vi "AE Paper.vi"(0 "error in (no error)":errorcluster, 1 "Message Queue in":T2, 2 "Events":dbl, 3 "Action Events":T1=enum."Init") -> (7 "error out":errorcluster, 9 "Event Increase":dbl)   [LabVIEW 2013, in "main.lvlib"]
uses:
  main.lvlib
  Components/Dependencies.llb/amc_Message Queue.ctl
  Components/Dependencies.llb/amc_Message.ctl
  <vilib>/FTP/util/Keyed Array.ctl
  Controls/Enum Paper Action Events.ctl
  Components/Dependencies.llb/TLB_Dependencies.lvlib
  <vilib>/FTP/NI_FTP.lvlib
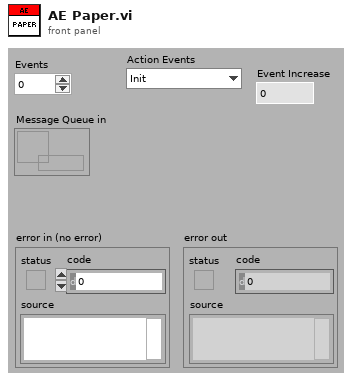
[diagram p1: front panel]
types:
  T1 = typedef "main.lvlib/Enum Paper Action Events.ctl" = enum16{"Paper State", "Init"}
  T2 = typedef "main.lvlib/TLB_Dependencies.lvlib/amc_Message Queue.ctl" = refnum<queue>
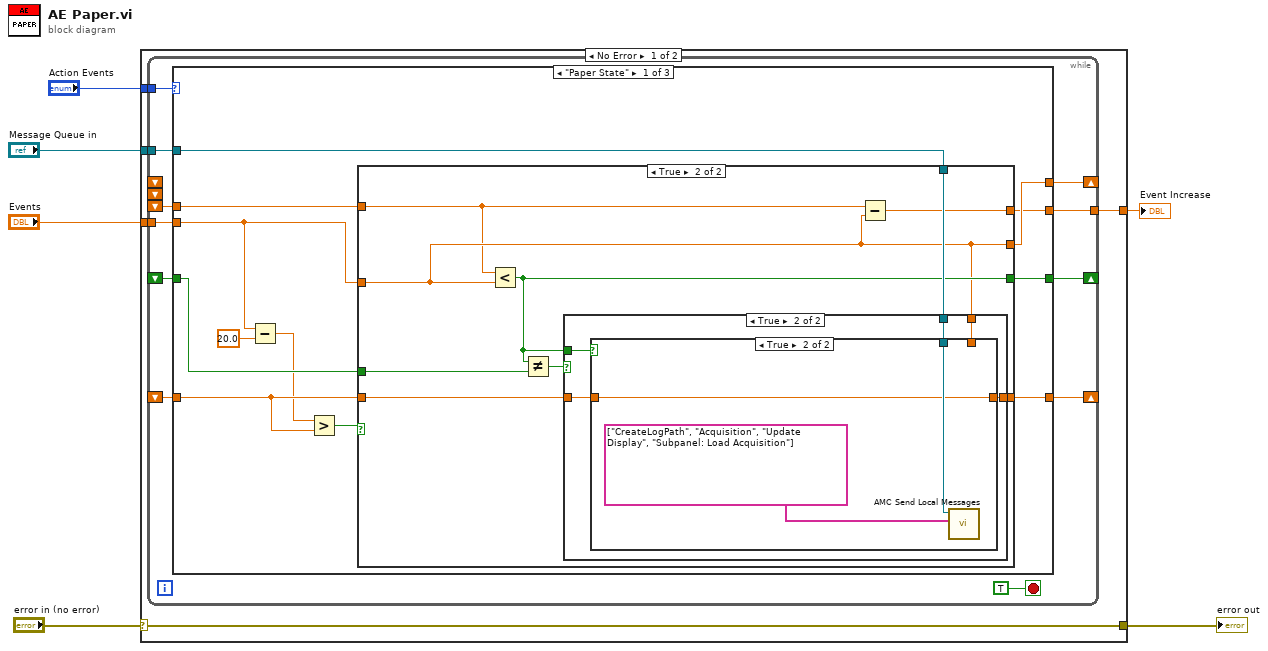
[diagram p0: block diagram]
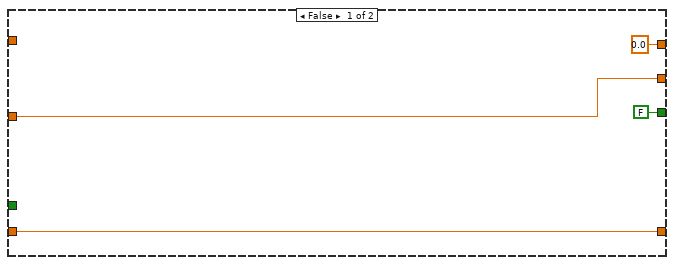
[diagram p2: hidden frame]
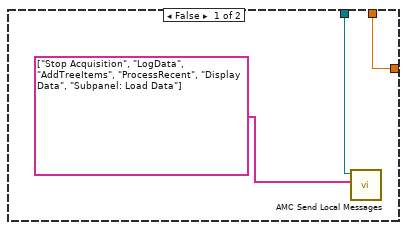
[diagram p4: hidden frame]
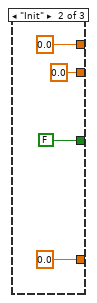
[diagram p5: hidden frame]
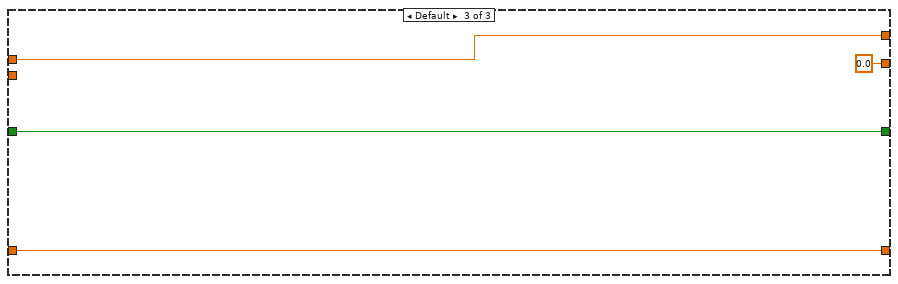
[diagram p6: hidden frame]
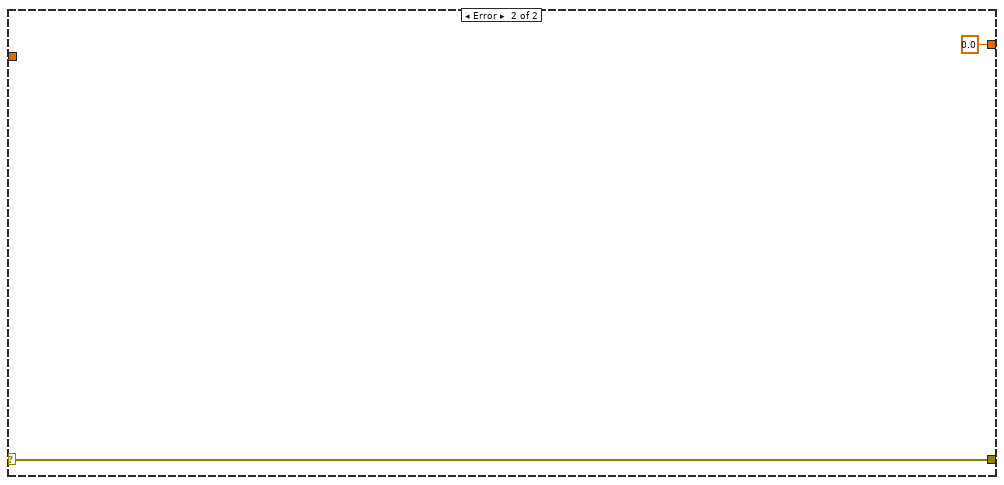
[diagram p7: hidden frame]
diagram:
  n1 = case shown="No Error" "error in (no error)" {
    selector: "error in (no error)" -> [w8 w69]
    tunnel: "Action Events" -> [w11 _]
    tunnel: "Message Queue in" -> [w10 _]
    tunnel: "Events" -> [w9 _]
    tunnel: [w8 w69] -> w2
    tunnel: [w7 0.0] -> w1
    frame No Error {
      n2 = while {
        tunnel: w11 -> [w21]
        tunnel: w10 -> [w20]
        shift-right: [w18] -> _
        shift-left: _ -> [_]
        tunnel: w9 -> [w19]
        shift-right: [w17] -> _
        shift-left: _ -> [w16]
        shift-left: _ -> [_]
        shift-left: _ -> [w15]
        shift-right: [w14] -> _
        shift-left: _ -> [w13]
        tunnel: [w12] -> w7
        stop <- TRUE stop-if-true
        n3 = case shown="\"Paper State\"" w21 {
          tunnel: w20 -> [w34 _ _]
          tunnel: w19 -> [w25 _ _]
          tunnel: [w29 0.0 ("Events") w66] -> w18
          tunnel: [w27 FALSE w67] -> w17
          tunnel: w16 -> [w28 _ w67]
          tunnel: w15 -> [w30 _ w66]
          tunnel: [w33 0.0 ("Events") w65] -> w14
          tunnel: w13 -> [w32 _ w65]
          tunnel: [w23 0.0 0.0] -> w12
          frame "Paper State" {
            n4 = Subtract(x=w25, y=20.0 ("x")) -> (x-y=w24:dbl)
            n5 = Greater?(x=w24, y=w32) -> (0:w31:bool)
            n6 = case shown="True" w31 {
              tunnel: w34 -> [_ w47]
              tunnel: [w36 w46] -> w33
              tunnel: w32 -> [w36 w45]
              tunnel: w30 -> [_ w40]
              tunnel: w25 -> [w38 w41]
              tunnel: [w38 w41] -> w29
              tunnel: w28 -> [_ w44]
              tunnel: [FALSE w42] -> w27
              tunnel: [0.0 w39] -> w23
              frame False {
              }
              frame True {
                n7 = Less?(x=w40, y=w41) -> (x < y?=w42:bool)
                n8 = Not Equal?(x=w42, y=w44) -> (x != y?=w43:bool)
                n9 = case shown="True" w43 {
                  tunnel: w47 -> [_ w53]
                  tunnel: [w48 w52] -> w46
                  tunnel: w45 -> [w48 w51]
                  tunnel: w42 -> [_ w50]
                  tunnel: w41 -> [_ w49]
                  frame False {
                  }
                  frame True {
                    n10 = case shown="True" w50 {
                      tunnel: w53 -> [w55 w58]
                      tunnel: [w54 w57] -> w52
                      tunnel: w51 -> [_ w57]
                      tunnel: w49 -> [w54 _]
                      frame False {
                        n11 = call "AMC Send Local Messages.vi"("Message Names"=string[] ["Stop Acquisition", "LogData", "AddTreeItems", "ProcessRecent", "Display Data", "Subpanel: Load Data"], "Message Queue in"=w55) -> ()  [unwired: 8 in, 2 out]
                      }
                      frame True {
                        n12 = call "AMC Send Local Messages.vi"("Message Names"=string[] ["CreateLogPath", "Acquisition", "Update Display", "Subpanel: Load Acquisition"], "Message Queue in"=w58) -> ()  [unwired: 8 in, 2 out]
                      }
                    }
                  }
                }
                n13 = Subtract(x=w40, y=w41) -> (x-y=w39:dbl)
              }
            }
          }
          frame "Init" {
          }
          frame Default {
          }
        }
      }
    }
    frame Error {
    }
  }
  "error out" <- w2
  "Event Increase" <- w1
